vi "ad discrete out64.vi"(7 "data":u64, 8 "error in (no error)":errorcluster, 9 "range":u64, 10 "cha":i32, 11 "adh":i32) -> (0 "error out":errorcluster, 3 "function return":i32)   [LabVIEW 2021, in "libad4.lvlib"]
doc: "LIBAD4 function: ad_discrete_out64 (int32_t adh, int32_t cha, uint64_t range, uint64_t data);\n\nSets a 64 bit output."
uses:
  <userlib>/libad4/libad4.lvlib
  <userlib>/libad4/libad4.dll
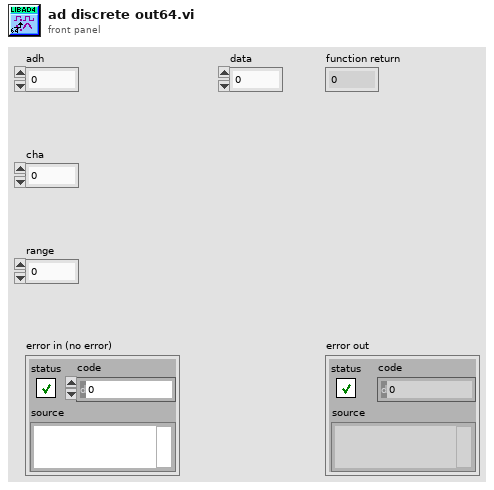
[diagram p1: front panel]
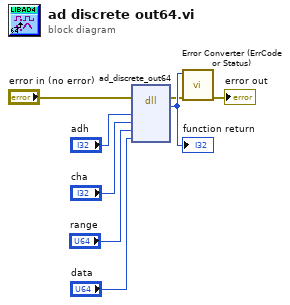
[diagram p0: block diagram]
diagram:
  n1 = dll-call lib="C:/Program Files/National Instruments/LabVIEW 2021/user.lib/libad4/libad4.*" fn="ad_discrete_out64"(error in="error in (no error)", "adh"="adh", "cha"="cha", "range"="range", "data"="data") -> (error out=w4:errorcluster, "return type"=w8:i32)  [unwired: 6 in, 1 out]
  "function return" <- w8
  n2 = call <userlib>:"Error Converter (ErrCode or Status).vi"("error in (no error)"=w4, "error code"=w8) -> ("error out"=→"error out":errorcluster)  [unwired: 9 in]
